vi "SendInitialOMFHTTPSPOSTS.vi"(0 "OMF Ingress URL":string, 1 "OMF Producer Token":string, 2 "Allow untrusted certificates?":bool=TRUE, 5 "OMF Static Type Message JSON":string, 7 "OMF Dynamic Type Message JSON":string, 9 "OMF Container Message JSON":string, 11 "OMF Static Type Instance Message JSON":string, 13 "OMF Link Message JSON":string) -> (14 "client handle out":T1, 15 "Reponse headers for initial OMF messages":string, 16 "Response body for initial OMF messages":string, 19 "error out":errorcluster)   [LabVIEW 2014]
uses:
  <vilib>/httpClient/ClientHandle.ctl
  <vilib>/httpClient/POSTBuffer.vi
  <vilib>/httpClient/LabVIEWHTTPClient.lvlib
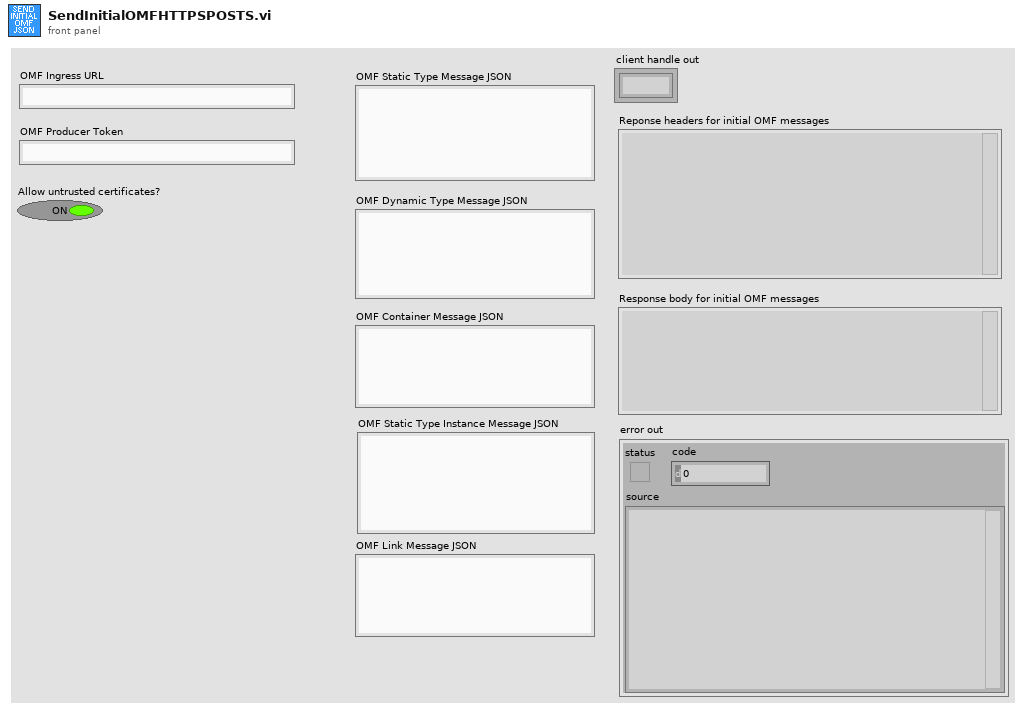
[diagram p1: front panel]
types:
  T1 = typedef "LabVIEWHTTPClient.lvlib/ClientHandle.ctl" = refnum<k1>
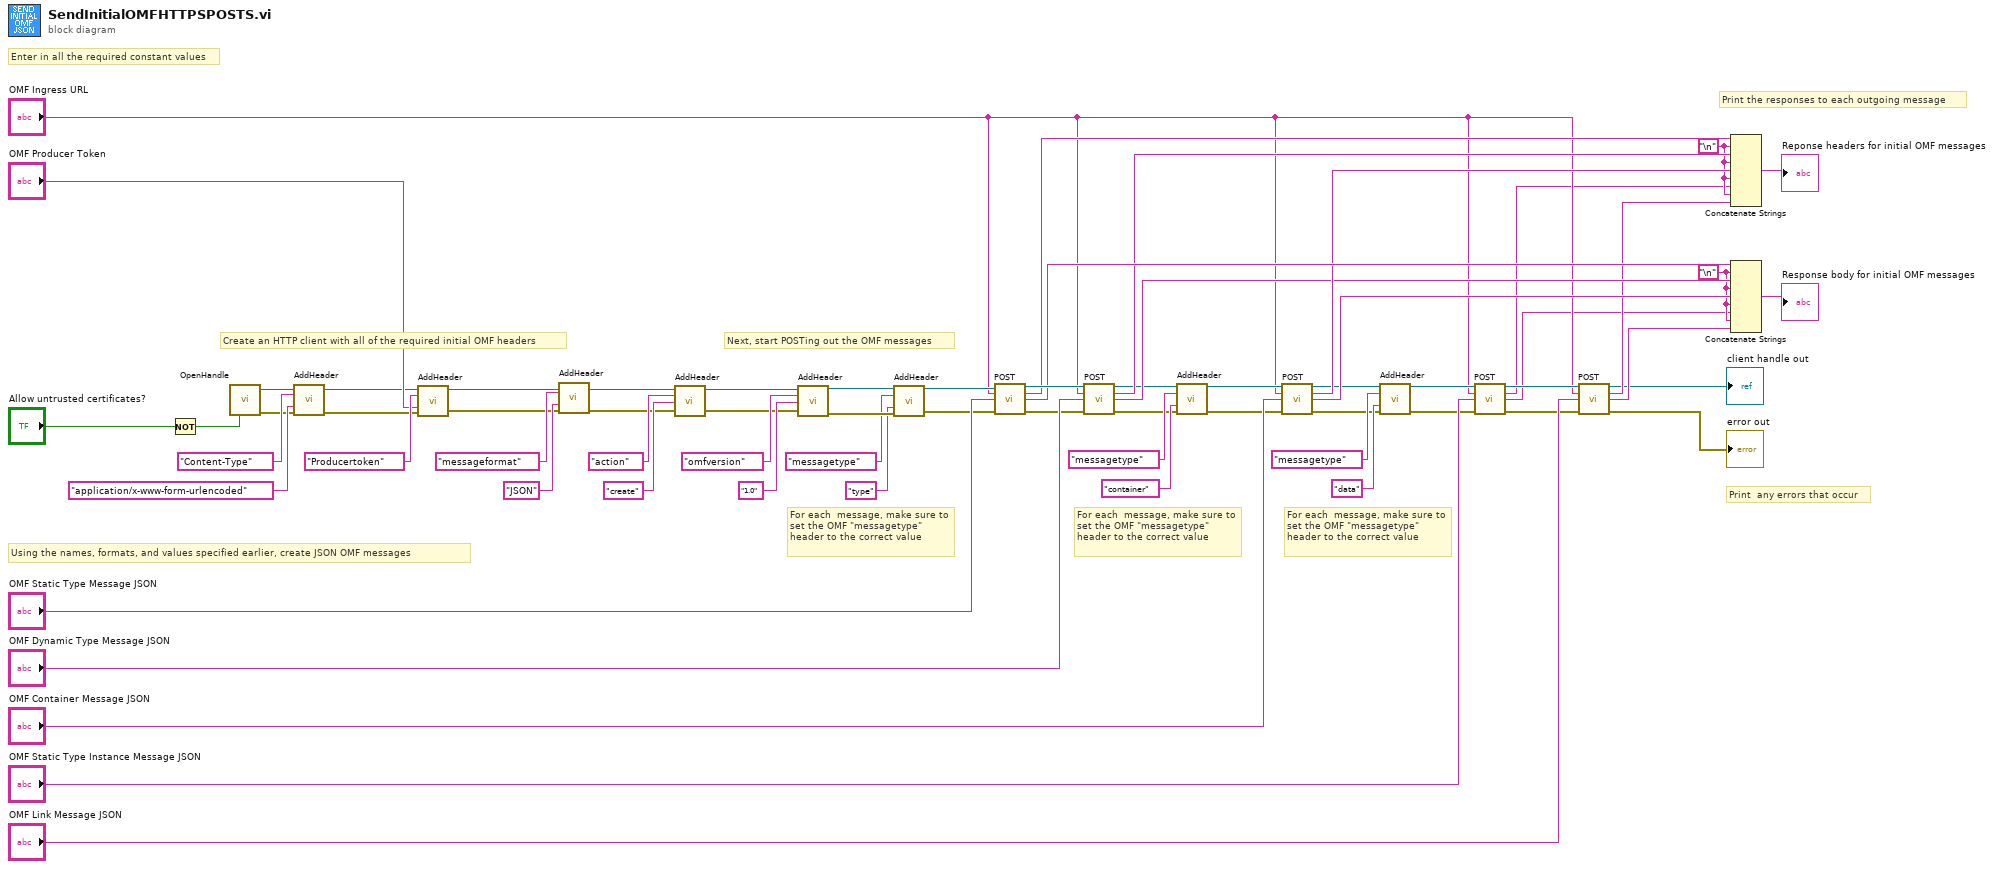
[diagram p0: block diagram]
diagram:
  w8 = "\n" ("string")
  w7 = "\n" ("string")
  # "Using the names, formats, and values specified earlier, create JSON OMF messages"
  # "For each  message, make sure to set the OMF \"messagetype\" header to the correct value"
  # "For each  message, make sure to set the OMF \"messagetype\" header to the correct value"
  # "For each  message, make sure to set the OMF \"messagetype\" header to the correct value"
  # "Print the responses to each outgoing message"
  # "Print  any errors that occur"
  # "Next, start POSTing out the OMF messages"
  # "Create an HTTP client with all of the required initial OMF headers"
  # "Enter in all the required constant values"
  n1 = Not(x="Allow untrusted certificates?") -> (.not. x?=w35:bool)
  n2 = call <vilib>:"OpenHandle.vi"("verify server(true)"=w35) -> ("client handle out"=w48:T1, "error out"=w47:errorcluster)  [unwired: 13 in]
  n3 = call <vilib>:"AddHeader.vi"("client handle"=w48, "header"="Content-Type", "value"="application/x-www-form-urlencoded", "error in (no error)"=w47) -> ("client handle out"=w50:T1, "error out"=w49:errorcluster)  [unwired: 10 in]
  n4 = call <vilib>:"AddHeader.vi"("client handle"=w50, "header"="Producertoken", "value"="OMF Producer Token", "error in (no error)"=w49) -> ("client handle out"=w52:T1, "error out"=w51:errorcluster)  [unwired: 10 in]
  n5 = call <vilib>:"AddHeader.vi"("client handle"=w52, "header"="messageformat", "value"="JSON", "error in (no error)"=w51) -> ("client handle out"=w62:T1, "error out"=w60:errorcluster)  [unwired: 10 in]
  n6 = call <vilib>:"AddHeader.vi"("client handle"=w62, "header"="action", "value"="create", "error in (no error)"=w60) -> ("client handle out"=w56:T1, "error out"=w57:errorcluster)  [unwired: 10 in]
  n7 = call <vilib>:"AddHeader.vi"("client handle"=w56, "header"="omfversion", "value"="1.0", "error in (no error)"=w57) -> ("client handle out"=w30:T1, "error out"=w27:errorcluster)  [unwired: 10 in]
  n8 = call <vilib>:"AddHeader.vi"("client handle"=w30, "header"="messagetype", "value"="type", "error in (no error)"=w27) -> ("client handle out"=w29:T1, "error out"=w28:errorcluster)  [unwired: 10 in]
  n9 = call-poly <vilib>:"POST.vi"("client handle"=w29, "url"="OMF Ingress URL", "buffer"="OMF Static Type Message JSON", "error in (no error)"=w28) -> ("client handle out"=w45:T1, "headers"=w40:string, "body"=w37:string, "error out"=w41:errorcluster)  [unwired: 8 in]
  n10 = call-poly <vilib>:"POST.vi"("client handle"=w45, "url"="OMF Ingress URL", "buffer"="OMF Dynamic Type Message JSON", "error in (no error)"=w41) -> ("client handle out"=w22:T1, "headers"=w33:string, "body"=w32:string, "error out"=w21:errorcluster)  [unwired: 8 in]
  n11 = call <vilib>:"AddHeader.vi"("client handle"=w22, "header"="messagetype", "value"="container", "error in (no error)"=w21) -> ("client handle out"=w20:T1, "error out"=w19:errorcluster)  [unwired: 10 in]
  n12 = call-poly <vilib>:"POST.vi"("client handle"=w20, "url"="OMF Ingress URL", "buffer"="OMF Container Message JSON", "error in (no error)"=w19) -> ("client handle out"=w16:T1, "headers"=w34:string, "body"=w31:string, "error out"=w15:errorcluster)  [unwired: 8 in]
  n13 = call <vilib>:"AddHeader.vi"("client handle"=w16, "header"="messagetype", "value"="data", "error in (no error)"=w15) -> ("client handle out"=w11:T1, "error out"=w13:errorcluster)  [unwired: 10 in]
  n14 = call-poly <vilib>:"POST.vi"("client handle"=w11, "url"="OMF Ingress URL", "buffer"="OMF Static Type Instance Message JSON", "error in (no error)"=w13) -> ("client handle out"=w10:T1, "headers"=w3:string, "body"=w4:string, "error out"=w12:errorcluster)  [unwired: 8 in]
  n15 = call-poly <vilib>:"POST.vi"("client handle"=w10, "url"="OMF Ingress URL", "buffer"="OMF Link Message JSON", "error in (no error)"=w12) -> ("client handle out"=→"client handle out":T1, "headers"=w6:string, "body"=w5:string, "error out"=→"error out":errorcluster)  [unwired: 8 in]
  n16 = Concatenate Strings "Concatenate Strings"(w40, w7, w33, w7, w34, w7, w3, w7, w6) -> (→"Reponse headers for initial OMF messages":string)
  n17 = Concatenate Strings "Concatenate Strings"(w37, w8, w32, w8, w31, w8, w4, w8, w5) -> (→"Response body for initial OMF messages":string)
